vi "Draw.vi"(8 "error in (no error)":errorcluster, 10 "2D Picture in":picture, 11 "Square in":refnum<class "Square.lvclass">) -> (0 "error out":errorcluster, 2 "2D Picture out":picture, 3 "Square out":refnum<class "Square.lvclass">)   [LabVIEW 2021, in "Picture2D.lvlib" / "Square.lvclass"]
uses:
  Square.lvclass
  Square.lvclass/Square.ctl
  Color/Color.lvclass
  Point/Point.lvclass
  Rectangle/Rectangle.lvclass
  Pen/Pen.lvclass
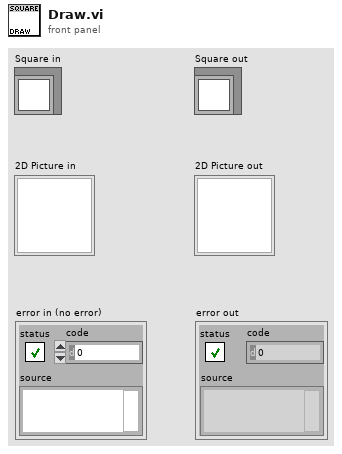
[diagram p1: front panel]
types:
  T1 = cluster{"Width":u16, "Style":enum32{"Solid", "Dash", "Dot", "DashDot", "DashDotDot"}}
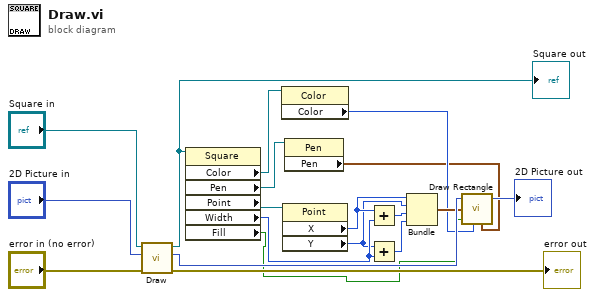
[diagram p0: block diagram]
diagram:
  n1 = call-parent "Draw.vi"("error in (no error)"="error in (no error)", "2D Picture in"="2D Picture in", "Rectangle in"="Square in") -> ("error out"=→"error out":errorcluster, "2D Picture out"=w15:picture, "Rectangle out"=w13:refnum<class "Square.lvclass">)  [unwired: 6 in]
  "Square out" <- w13
  n2 = property class="Square"(reference=w13) -> ("Color"=w5:refnum<class "Color.lvclass">, "Pen"=w3:refnum<class "Pen.lvclass">, "Point"=w12:refnum<class "Point.lvclass">, "Width"=w8:i16, "Fill"=w1:bool)  [unwired: 1 in, 2 out]
  n3 = property class="Color"(reference=w5) -> ("Color"=w4:u32)  [unwired: 1 in, 2 out]
  n4 = property class="Point"(reference=w12) -> ("X"=w11:i16, "Y"=w7:i16)  [unwired: 1 in, 2 out]
  n5 = property class="Pen"(reference=w3) -> ("Pen"=w2:T1)  [unwired: 1 in, 2 out]
  n6 = Add(x=w11, y=w8) -> (x+y=w9:i16)
  n7 = Add(x=w7, y=w8) -> (x+y=w6:i16)
  n8 = Bundle("X"=w11, "Y"=w7, w9, w6) -> (w10:cluster{"X":i16, "Y":i16, i16, i16})  [unwired: 1 in]
  n9 = call <vilib>:"Draw Rectangle.vi"("picture"=w15, "rect"=w10, "fill?(F)"=w1, "color(black)"=w4, "pen"=w2) -> ("new picture"=→"2D Picture out":picture)  [unwired: 4 in]
